vi "DrawHamiltonianCycle.vi"(8 "error in (no error)":errorcluster, 11 "path to tmx-file (created with Tiles2D)":path=path "/home/lvuser/natinst/bin/data/maps/HamiltonianCycle.tmx") -> (0 "error out":errorcluster, 1 "startpos":cluster{i32, i32}, 2 "Hamilton2D":u32[][](array[numeric]), 3 "Hamilton1D":cluster{i32, i32}[](array[cluster]))   [LabVIEW 2019, in "RT_Game.lvlib" / "AI_Snake.lvclass"]
uses:
  AI_Snake.lvclass
  Direction.ctl
  RT_Game.lvlib
  Engine/Engine.lvclass
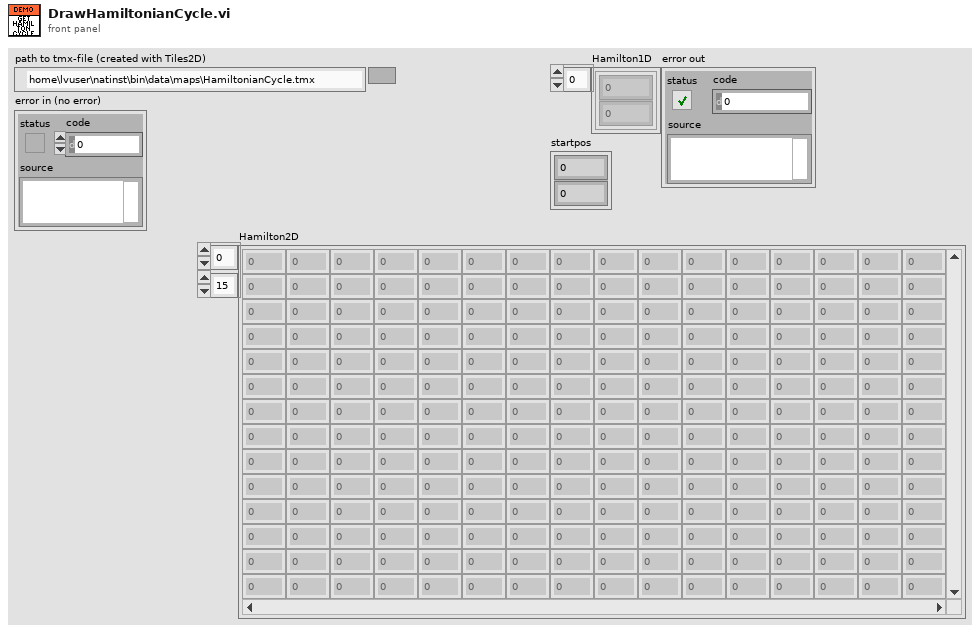
[diagram p1: front panel]
types:
  T1 = typedef "RT_Game.lvlib/Direction.ctl" = enum16{"none", "Both", "left", "right", "up", "down"}
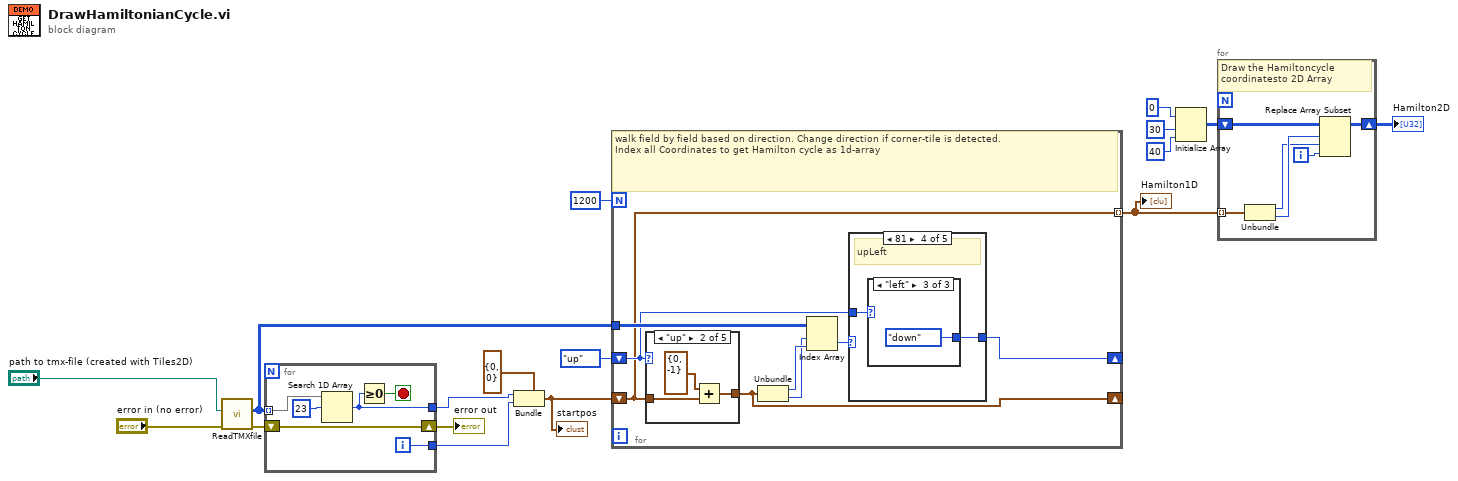
[diagram p0: block diagram]
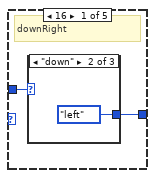
[diagram p2: hidden frame]
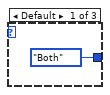
[diagram p3: hidden frame]
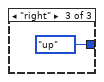
[diagram p4: hidden frame]
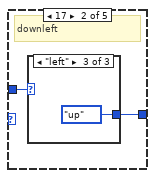
[diagram p5: hidden frame]
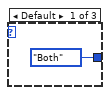
[diagram p6: hidden frame]
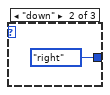
[diagram p7: hidden frame]
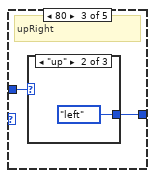
[diagram p8: hidden frame]
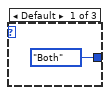
[diagram p9: hidden frame]
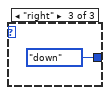
[diagram p10: hidden frame]
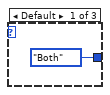
[diagram p11: hidden frame]
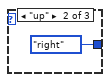
[diagram p12: hidden frame]
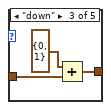
[diagram p15: hidden frame]
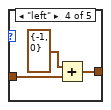
[diagram p16: hidden frame]
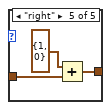
[diagram p17: hidden frame]
diagram:
  n1 = call "ReadTMXfile.vi"("error in (no error)"="error in (no error)", "path to tmx-file (created with Tiles2D)"="path to tmx-file (created with Tiles2D)") -> ("error out"=w10:errorcluster, "Tilenumbers"=w8:u32[][])  [unwired: 8 in]
  n2 = for {
    tunnel: [w23] -> w13
    tunnel: [w21] -> w12
    shift-right: [w20] -> w1
    shift-left: w10 -> [w20]
    tunnel: w8 -> [w19] mode=indexing
    i -> [w21]
    stop <- w22 stop-if-true
    n3 = Search 1D Array(1D array=w19, element=u32 23) -> (index of element=w23:i32)  [unwired: 1 in]
    n4 = Greater Or Equal To 0?(x=w23) -> (x >= 0?=w22:bool)
  }
  "error out" <- w1
  n5 = Bundle(cluster=cluster{i32, i32} {0, 0}, w13, w12) -> (w11:cluster{i32, i32})
  "startpos" <- w11
  n6 = for {
    N: 1200 -> [_]
    shift-right: [w27] -> _
    shift-left: Direction."up" ("Direction") -> [w25]
    shift-right: [w30] -> _
    shift-left: w11 -> [w24]
    tunnel: w8 -> [w31]
    tunnel: [w24] -> w7 mode=indexing
    # "walk field by field based on direction. Change direction if corner-tile is detected.\nIndex all Coordinates to get Hamilton cycle as 1d-array"
    n7 = case shown="\"up\"" w25 {
      tunnel: w24 -> [w53 w56 w59 w62 w65]
      tunnel: [w53 w55 w58 w61 w64] -> w30
      frame Default {
      }
      frame "up" {
        n8 = Add(x=cluster{i32, i32} {0, -1}, y=w56) -> (x+y=w55:cluster{i32, i32})
      }
      frame "down" {
        n9 = Add(x=cluster{i32, i32} {0, 1}, y=w59) -> (x+y=w58:cluster{i32, i32})
      }
      frame "left" {
        n10 = Add(x=cluster{i32, i32} {-1, 0}, y=w62) -> (x+y=w61:cluster{i32, i32})
      }
      frame "right" {
        n11 = Add(x=cluster{i32, i32} {1, 0}, y=w65) -> (x+y=w64:cluster{i32, i32})
      }
    }
    n12 = Unbundle(w30) -> (w29:i32, w28:i32)
    n13 = Index Array(array=w31, index (row)=w28, index (col)=w29) -> (element=w26:u32)
    n14 = case shown="81" w26 {
      tunnel: [w33 w38 w43 w48 w52] -> w27
      tunnel: w25 -> [w32 w37 w42 w47 w52]
      frame 16 {
        # "downRight"
        n15 = case shown="\"down\"" w32 {
          tunnel: [Direction."Both" ("Direction") Direction."left" ("Direction") Direction."up" ("Direction")] -> w33
          frame Default {
          }
          frame "down" {
          }
          frame "right" {
          }
        }
      }
      frame 17 {
        # "downleft"
        n16 = case shown="\"left\"" w37 {
          tunnel: [Direction."Both" ("Direction") Direction."right" ("Direction") Direction."up" ("Direction")] -> w38
          frame Default {
          }
          frame "down" {
          }
          frame "left" {
          }
        }
      }
      frame 80 {
        # "upRight"
        n17 = case shown="\"up\"" w42 {
          tunnel: [Direction."Both" ("Direction") Direction."left" ("Direction") Direction."down" ("Direction")] -> w43
          frame Default {
          }
          frame "up" {
          }
          frame "right" {
          }
        }
      }
      frame 81 {
        # "upLeft"
        n18 = case shown="\"left\"" w47 {
          tunnel: [Direction."Both" ("Direction") Direction."right" ("Direction") Direction."down" ("Direction")] -> w48
          frame Default {
          }
          frame "up" {
          }
          frame "left" {
          }
        }
      }
      frame 84, 85, Default {
      }
    }
  }
  "Hamilton1D" <- w7
  n19 = Initialize Array(u32 0 ("element"), 30 ("dimension size"), 40 ("dimension size")) -> (w3:u32[][])
  n20 = for {
    tunnel: w7 -> [w68] mode=indexing
    shift-right: [w70] -> w2
    shift-left: w3 -> [w71]
    i -> [w69]
    # "Draw the Hamiltoncycle\ncoordinatesto 2D Array"
    n21 = Unbundle(w68) -> (w66:i32, w67:i32)
    n22 = Replace Array Subset(array=w71, new element=w69, index (row)=w67, index (col)=w66) -> (w70:u32[][])
  }
  "Hamilton2D" <- w2
